vi "DSF.Shared.Configuration.Transfer.Errors.vi"   [LabVIEW 2017, in "DSF.Shared.lvlib" / "DSF.Shared.Configuration.Transfer.lvclass"]
uses:
  DSF.Shared.Configuration.Transfer.lvclass
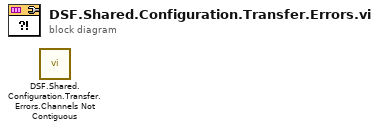
[diagram p0: block diagram]
diagram:
  n1 = call "DSF.Shared.Configuration.Transfer.Errors.Channels Not Contiguous.vi"() -> ()  [unwired: 10 in, 2 out]
